vi "atm-machine.vi"() -> ()   [LabVIEW 2017]
panel:
  in  "LOGIN":bool
  out "act 6":string
  out "act 5":string
  out "act 4":string
  out "act 3":string
  out "act 1":string
  out "act 2":string
  in  "but6":bool
  in  "but5":bool
  in  "but4":bool
  in  "but3":bool
  in  "but2":bool
  in  "but1":bool
  in  "Enter PIN":string="0000"
  out "ATM Screen":string
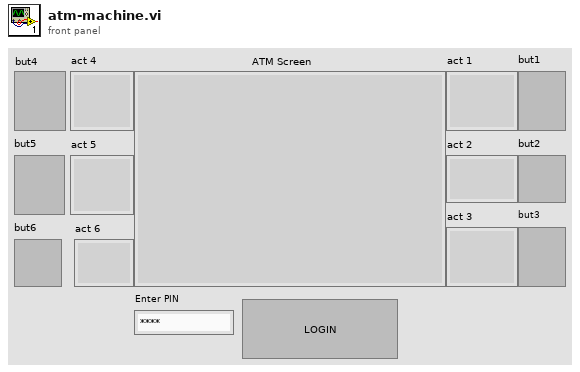
[diagram p1: front panel]
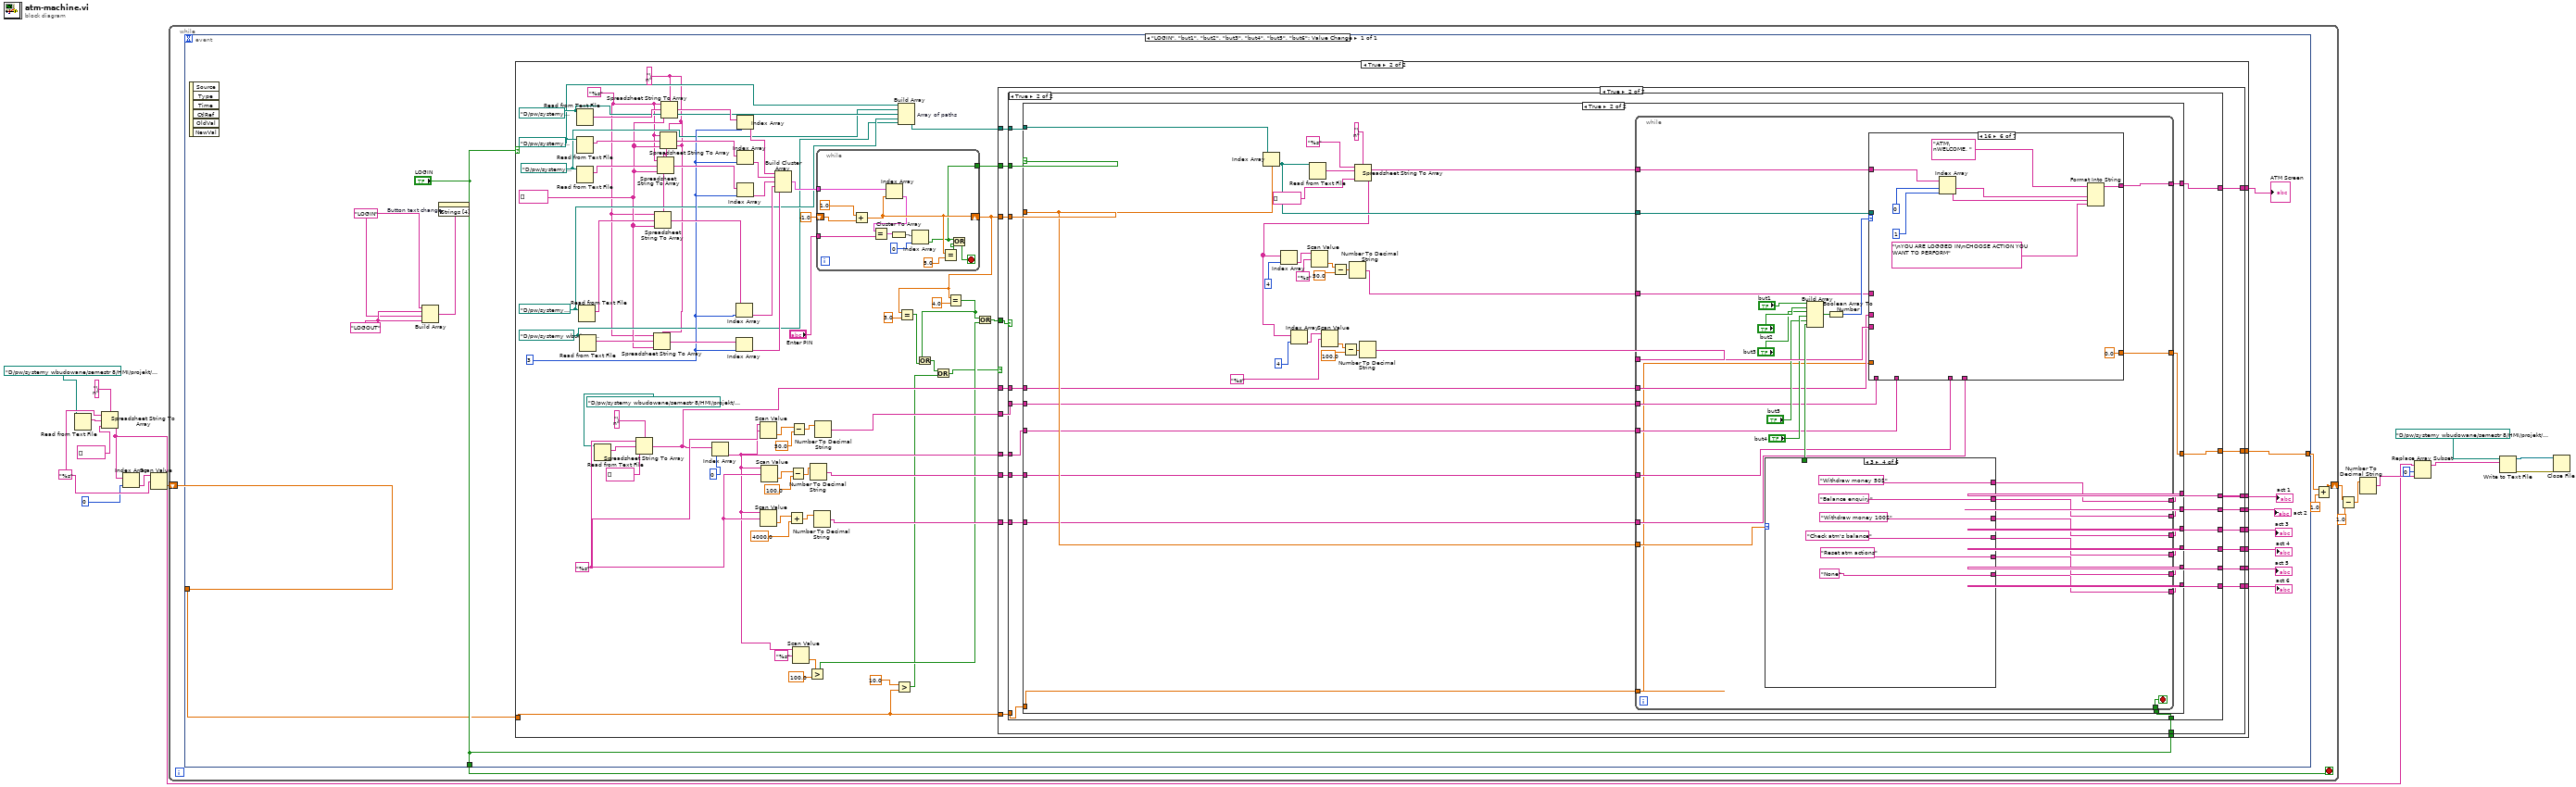
[diagram p0: block diagram]
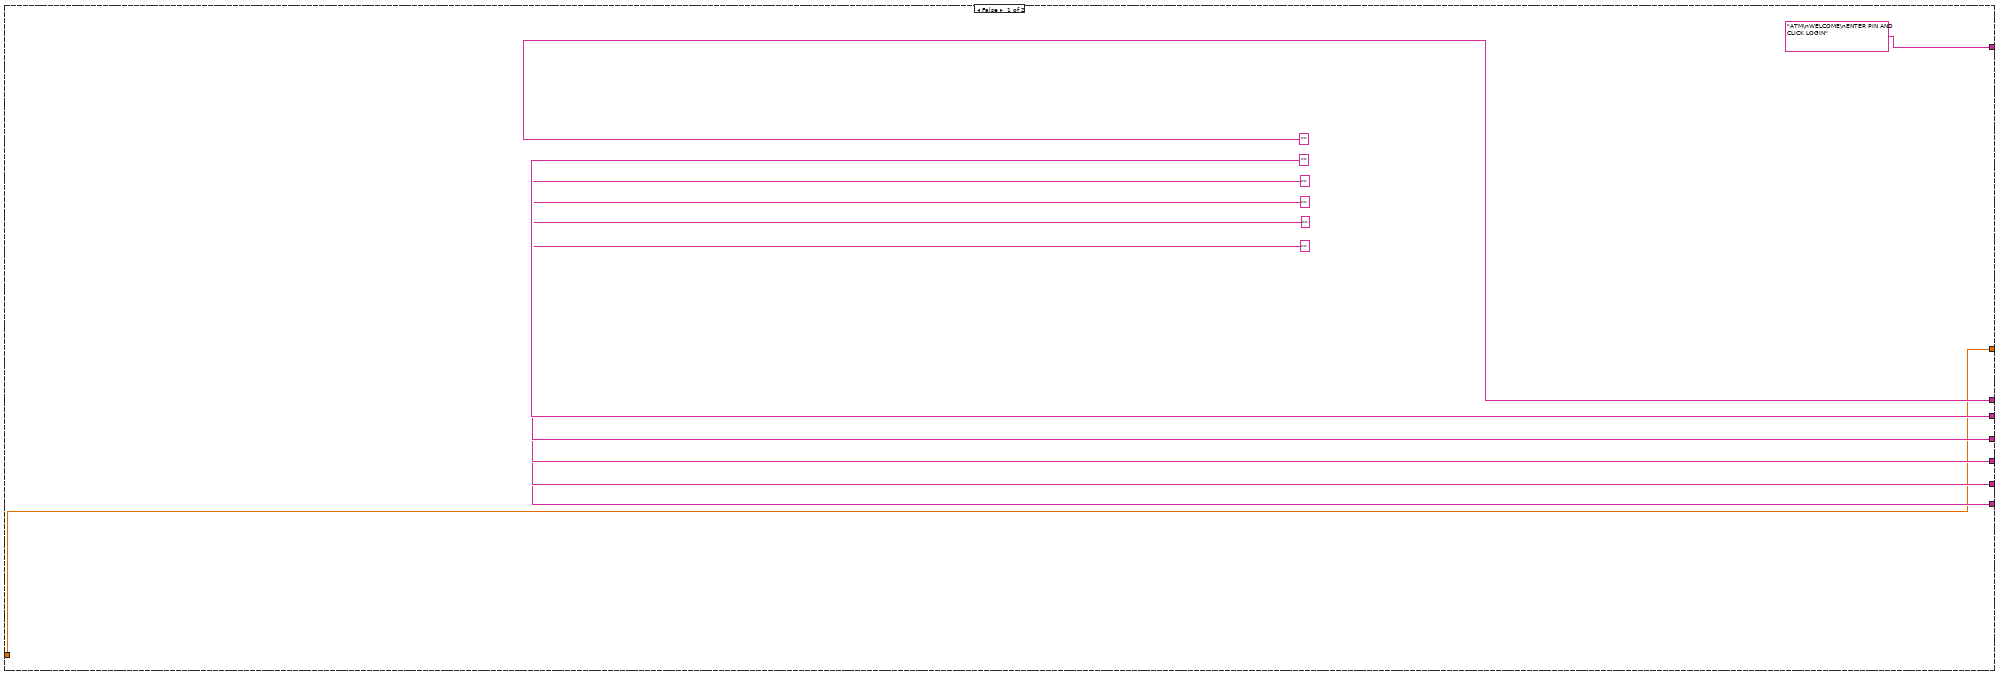
[diagram p2: hidden frame]
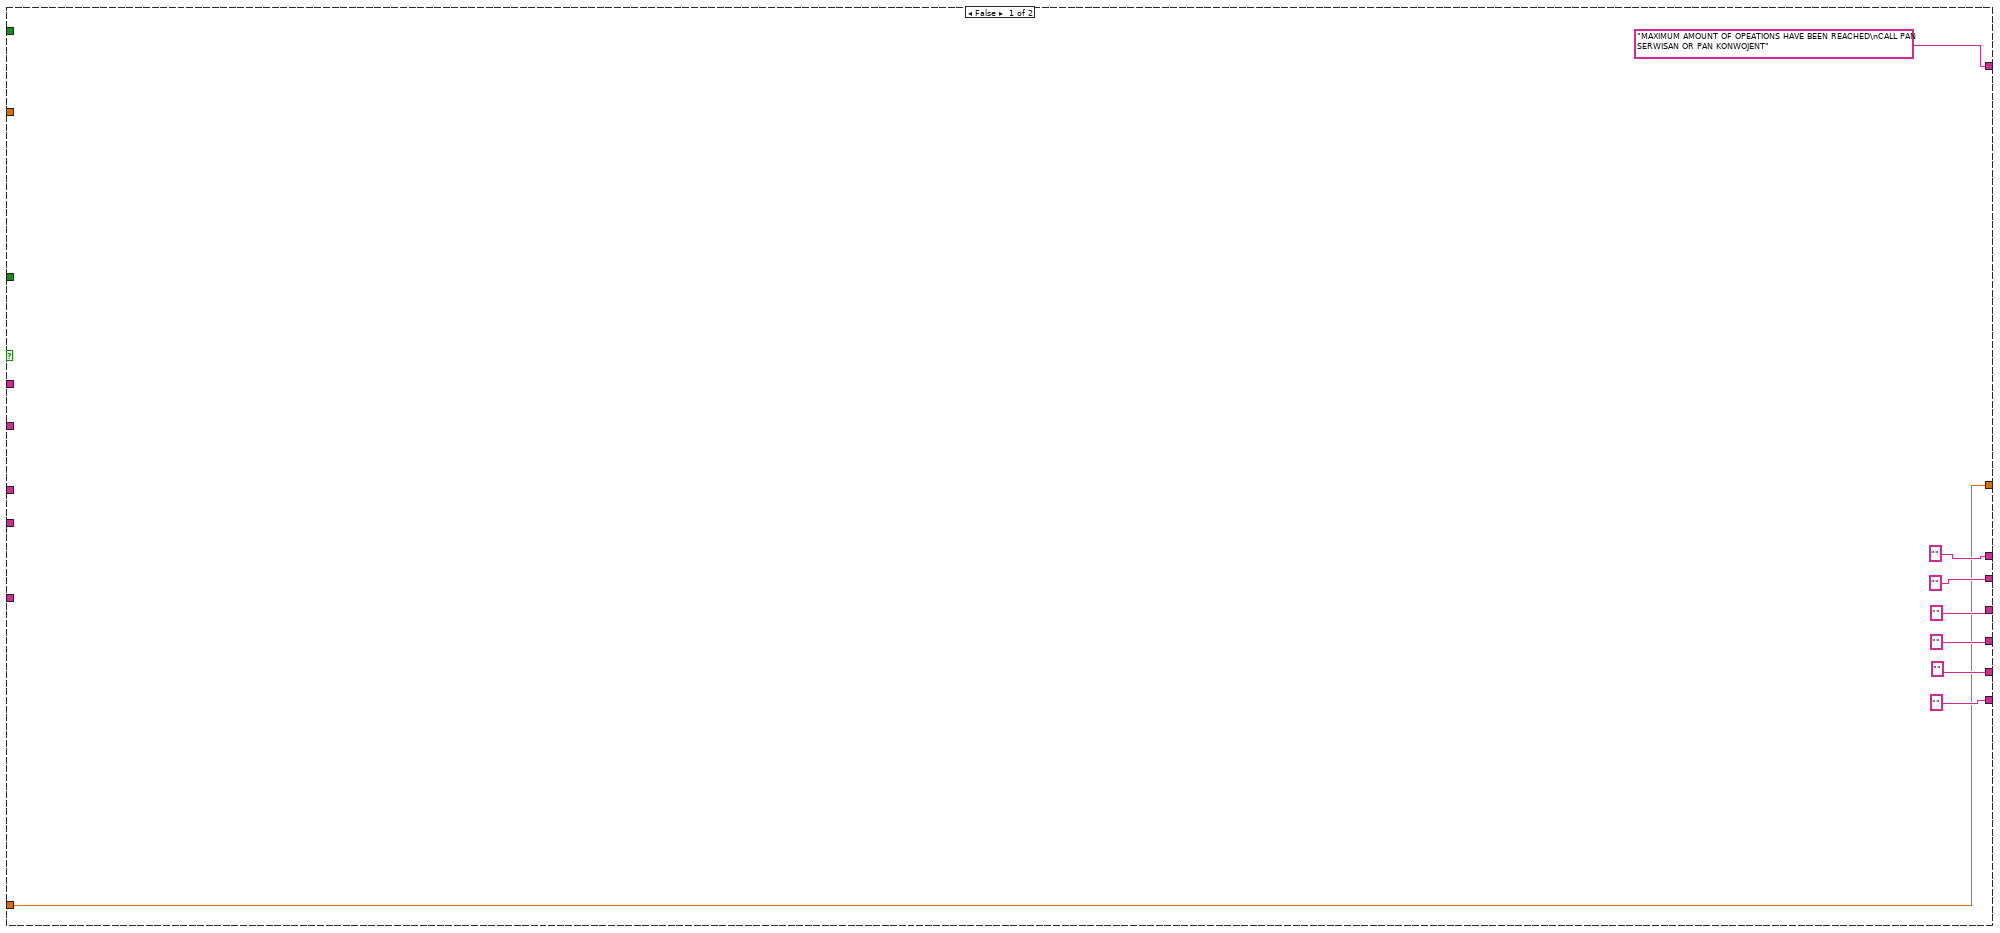
[diagram p3: hidden frame]
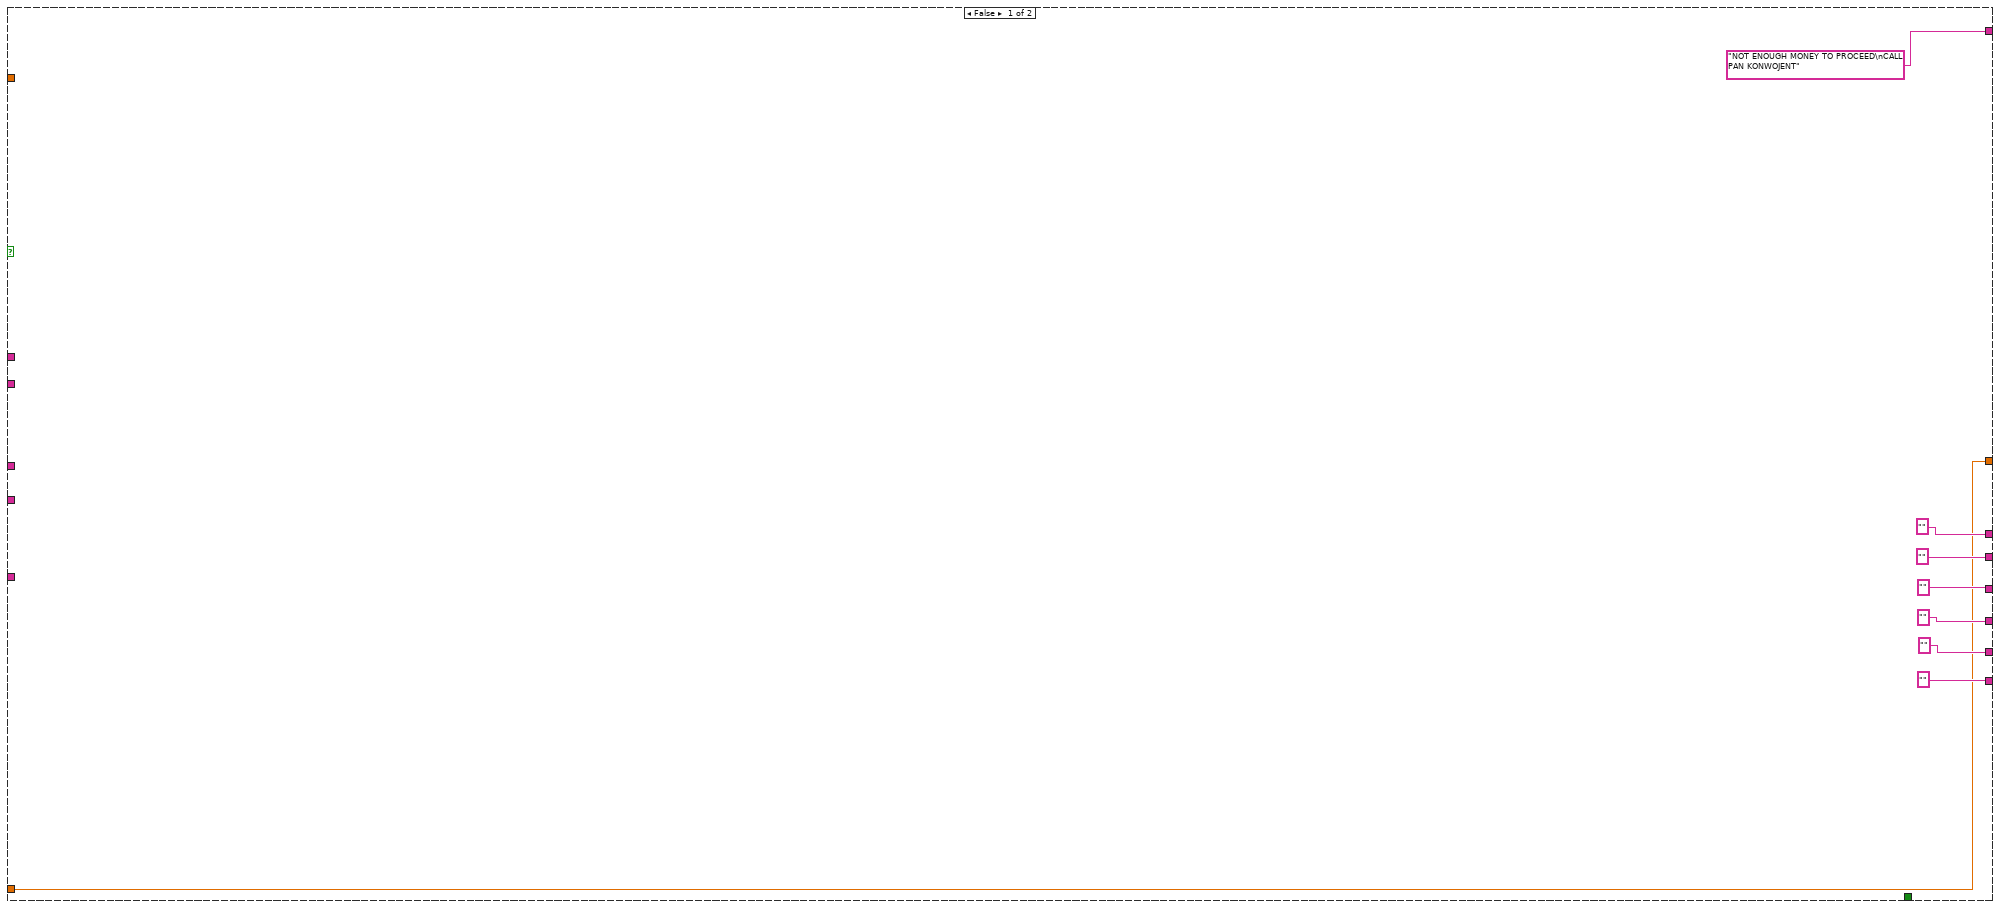
[diagram p4: hidden frame]
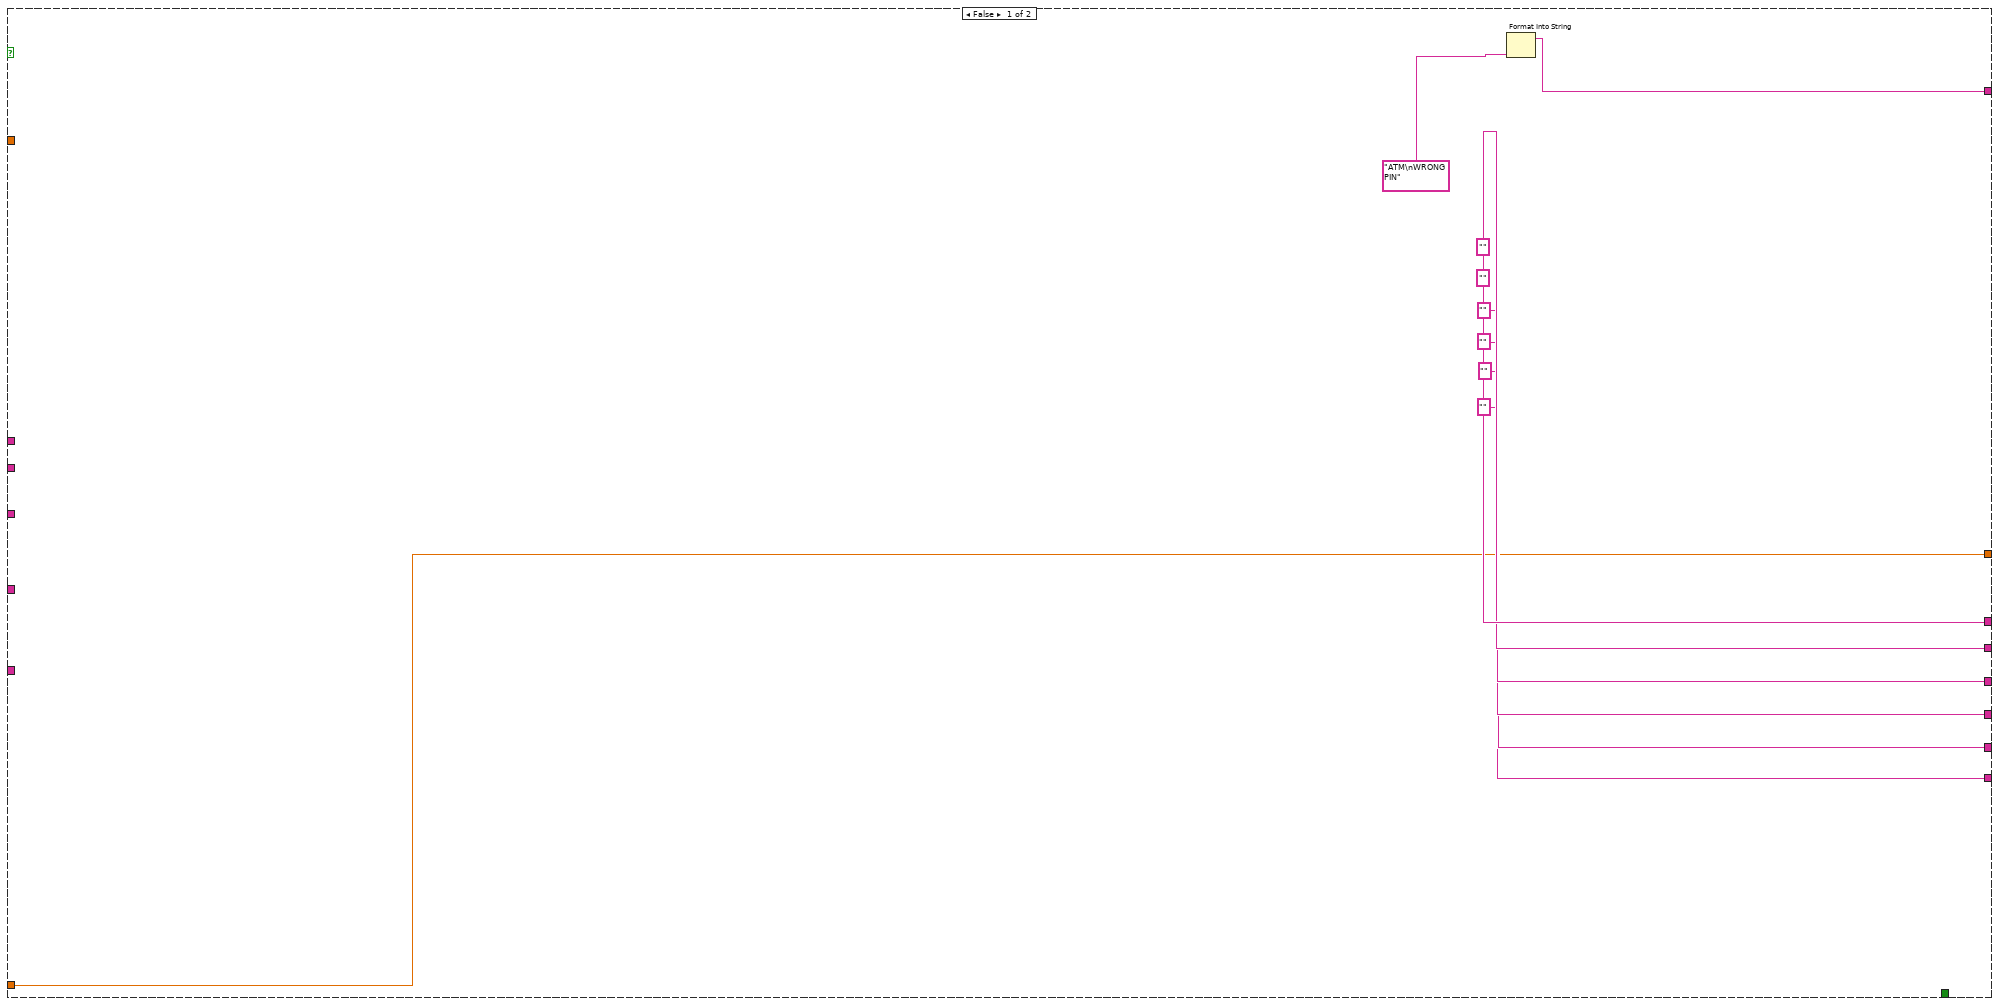
[diagram p5: hidden frame]
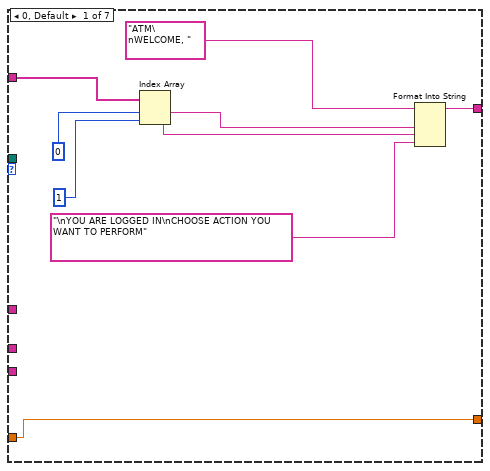
[diagram p6: hidden frame]
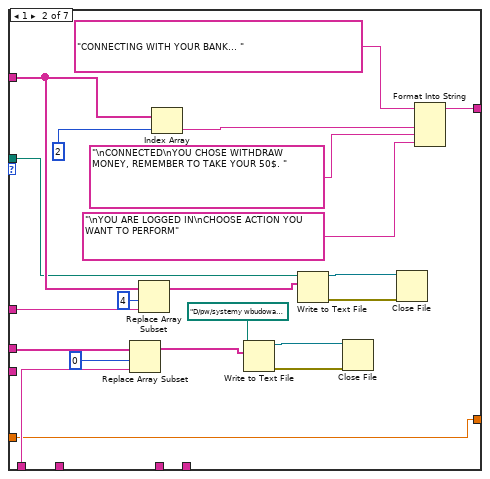
[diagram p7: hidden frame]
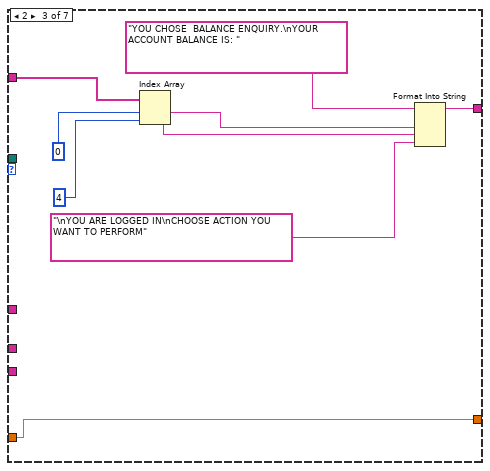
[diagram p8: hidden frame]
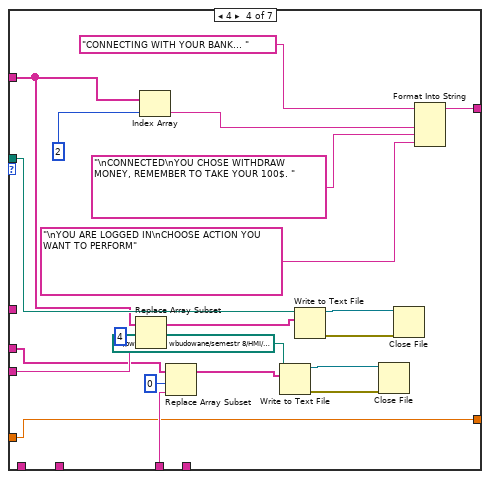
[diagram p9: hidden frame]
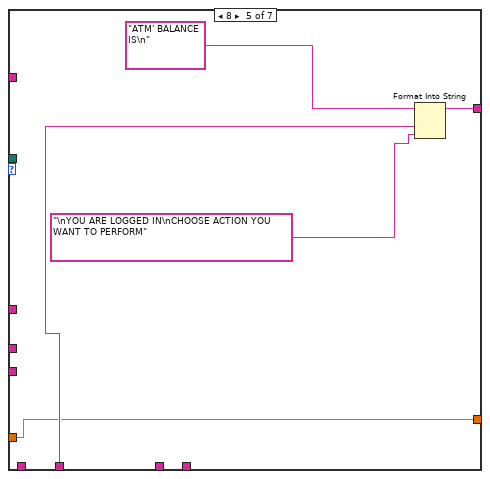
[diagram p10: hidden frame]
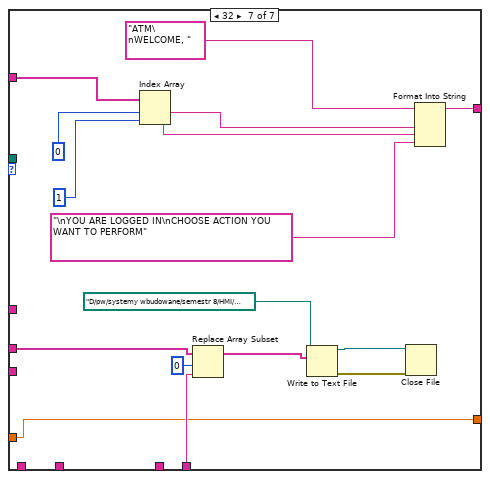
[diagram p11: hidden frame]
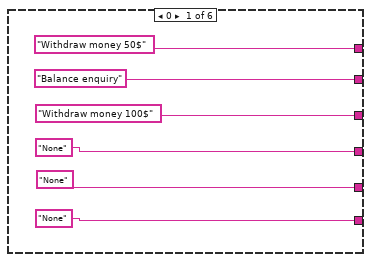
[diagram p12: hidden frame]
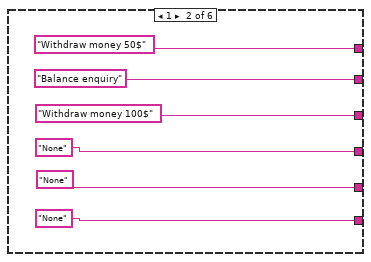
[diagram p13: hidden frame]
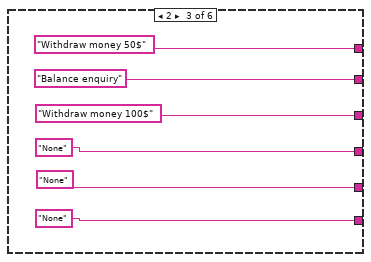
[diagram p14: hidden frame]
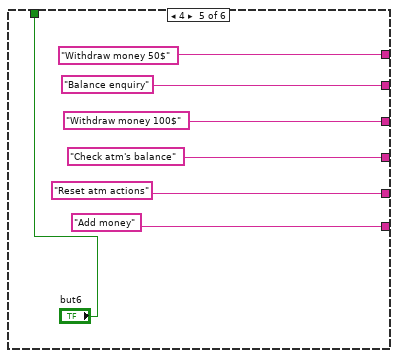
[diagram p15: hidden frame]
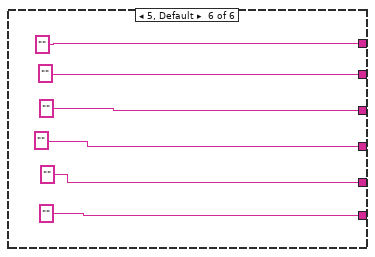
[diagram p16: hidden frame]
diagram:
  w16 = "%s" ("format string")
  n1 = Read from Text File(file (use dialog)=path "D:/pw/systemy wbudowane/semestr 8/HMI/projekt/bankomat-iteracje.txt") -> (text=w17:string)  [unwired: 3 in, 3 out]
  n2 = Spreadsheet String To Array(delimiter (Tab)="\n", format string=w16, spreadsheet string=w17, array type (2D Dbl)=string[] [] ("Array")) -> (array=w6:string[])
  n3 = Index Array "Index Array"(array=w6, index=0) -> (element=w18:string)
  n4 = Scan Value(string=w18, format string=w16) -> (value=w11:dbl)  [unwired: 1 in, 1 out]
  n5 = while {
    shift-right: [w20] -> w3
    shift-left: w11 -> [w22]
    stop <- w23 stop-if-true
    n6 = event shown="[0] \"LOGIN\", \"but1\", \"but2\", \"but3\", \"but4\", \"but5\", \"but6\": Value Change" {
      selector: _ -> [_]
      dyn-events: _ -> [_]
      timeout: _ -> [_]
      tunnel: ["LOGIN"] -> w23
      tunnel: [w25] -> w19
      tunnel: w22 -> [w24]
      event "LOGIN", "but1", "but2", "but3", "but4", "but5", "but6": Value Change {
        w29 = "LOGOUT" ("new ON text")
        w28 = "LOGIN" ("new OFF text")
        n7 = event-data() -> ()  [unwired: 1 in, 6 out]
        n8 = Build Array(w28, w29, w28, w29) -> (w30:string[])
        n9 = property on="Button text change" class="Bool (strict)"("Strings [4]"=w30) -> ()  [unwired: 2 in, 2 out]
        n10 = case shown="True" "LOGIN" {
          tunnel: ["" w93] -> w36
          tunnel: ["" w94] -> w35
          tunnel: ["" w95] -> w34
          tunnel: ["" w96] -> w33
          tunnel: ["" w98] -> w32
          tunnel: ["" w97] -> w31
          tunnel: "LOGIN" -> [_ w85]
          tunnel: ["ATM\nWELCOME\nENTER PIN AND CLICK LOGIN" w84] -> w26
          tunnel: [w37 w80] -> w25
          tunnel: w24 -> [w37 w51]
          frame False {
          }
          frame True {
            w67 = "%s" ("format string")
            w81 = "\n" ("delimiter (Tab)")
            w82 = "%s" ("format string")
            w106 = 3 ("index (row)")
            w83 = string[] [] ("Array")
            w87 = path "D:/pw/systemy wbudowane/semestr 8/HMI/projekt/konwojent.txt" ("file (use dialog)")
            w88 = path "D:/pw/systemy wbudowane/semestr 8/HMI/projekt/serwisant.txt" ("file (use dialog)")
            w89 = path "D:/pw/systemy wbudowane/semestr 8/HMI/projekt/klient-3.txt" ("file (use dialog)")
            w90 = path "D:/pw/systemy wbudowane/semestr 8/HMI/projekt/klient-2.txt" ("file (use dialog)")
            w91 = path "D:/pw/systemy wbudowane/semestr 8/HMI/projekt/klient-1.txt" ("file (use dialog)")
            n11 = Read from Text File(file (use dialog)=w90) -> (text=w114:string)  [unwired: 3 in, 3 out]
            n12 = Read from Text File(file (use dialog)=w89) -> (text=w113:string)  [unwired: 3 in, 3 out]
            n13 = Read from Text File(file (use dialog)=w91) -> (text=w117:string)  [unwired: 3 in, 3 out]
            n14 = Read from Text File(file (use dialog)=w88) -> (text=w112:string)  [unwired: 3 in, 3 out]
            n15 = Read from Text File(file (use dialog)=w87) -> (text=w111:string)  [unwired: 3 in, 3 out]
            n16 = Read from Text File(file (use dialog)=path "D:/pw/systemy wbudowane/semestr 8/HMI/projekt/bankomat-stan-konta.txt") -> (text=w78:string)  [unwired: 3 in, 3 out]
            n17 = Spreadsheet String To Array(delimiter (Tab)="\n", format string=w67, spreadsheet string=w78, array type (2D Dbl)=string[] [] ("Array")) -> (array=w61:string[])
            n18 = Spreadsheet String To Array(delimiter (Tab)=w81, format string=w82, spreadsheet string=w111, array type (2D Dbl)=w83) -> (array=w107:string[])
            n19 = Spreadsheet String To Array(delimiter (Tab)=w81, format string=w82, spreadsheet string=w112, array type (2D Dbl)=w83) -> (array=w108:string[])
            n20 = Spreadsheet String To Array(delimiter (Tab)=w81, format string=w82, spreadsheet string=w113, array type (2D Dbl)=w83) -> (array=w109:string[])
            n21 = Spreadsheet String To Array(delimiter (Tab)=w81, format string=w82, spreadsheet string=w114, array type (2D Dbl)=w83) -> (array=w110:string[])
            n22 = Spreadsheet String To Array(delimiter (Tab)=w81, format string=w82, spreadsheet string=w117, array type (2D Dbl)=w83) -> (array=w116:string[])
            n23 = Index Array "Index Array"(array=w61, index=0) -> (element=w60:string)
            n24 = Index Array "Index Array"(array=w108, index=w106) -> (element=w103:string)
            n25 = Index Array "Index Array"(array=w107, index=w106) -> (element=w102:string)
            n26 = Index Array "Index Array"(array=w109, index=w106) -> (element=w104:string)
            n27 = Index Array "Index Array"(array=w116, index=w106) -> (element=w115:string)
            n28 = Index Array "Index Array"(array=w110, index=w106) -> (element=w105:string)
            n29 = Scan Value(string=w60, format string=w67) -> (value=w74:dbl)  [unwired: 1 in, 1 out]
            n30 = Scan Value(string=w60, format string=w67) -> (value=w72:dbl)  [unwired: 1 in, 1 out]
            n31 = Scan Value(string=w60, format string=w67) -> (value=w73:dbl)  [unwired: 1 in, 1 out]
            n32 = Build Cluster Array "Build Cluster Array"(w115, w105, w104, w103, w102) -> (w101:cluster{"String":string}[])
            n33 = Add(x=w74, y=4000.0) -> (x+y=w77:dbl)
            n34 = Subtract(x=w73, y=100.0) -> (x-y=w76:dbl)
            n35 = Subtract(x=w72, y=50.0) -> (x-y=w75:dbl)
            n36 = Scan Value(string=w60, format string="%s") -> (value=w79:dbl)  [unwired: 1 in, 1 out]
            n37 = Greater?(x=w79, y=100.0) -> (0:w56:bool)
            n38 = Number To Decimal String(number=w76) -> (decimal integer string=w58:string)  [unwired: 1 in]
            n39 = Number To Decimal String(number=w77) -> (decimal integer string=w59:string)  [unwired: 1 in]
            n40 = Number To Decimal String(number=w75) -> (decimal integer string=w57:string)  [unwired: 1 in]
            n41 = while {
              tunnel: w101 -> [w384]
              shift-right: [w380] -> w53
              shift-left: -1.0 -> [w382]
              tunnel: "Enter PIN" -> [w379]
              tunnel: [w372] -> w92
              stop <- w373 stop-if-true
              n42 = Add(x=1.0 ("y"), y=w382) -> (x+y=w380:dbl)
              n43 = Index Array "Index Array"(array=w384, index=w380) -> (element=w378:cluster{"String":string})
              n44 = Equal?(x=w378, y=w379) -> (x = y?=w377:cluster{"String":bool})
              n45 = Cluster To Array(cluster=w377) -> (array=w376:bool[])
              n46 = Index Array "Index Array"(array=w376, index=0) -> (element=w372:bool)
              n47 = Equal?(x=w380, y=5.0 ("x")) -> (x = y?=w374:bool)
              n48 = Or(x=w372, y=w374) -> (x .or. y?=w373:bool)
            }
            n49 = Greater?(x=10.0, y=w51) -> (0:w49:bool)
            n50 = Build Array "Array of paths"(w91, w90, w89, w88, w87) -> (w86:path[])
            n51 = Equal?(x=w53, y=3.0) -> (x = y?=w46:bool)
            n52 = Equal?(x=w53, y=4.0) -> (x = y?=w45:bool)
            n53 = Or(x=w45, y=w46) -> (x .or. y?=w47:bool)
            n54 = Or(x=w47, y=w49) -> (x .or. y?=w48:bool)
            n55 = Or(x=w45, y=w56) -> (x .or. y?=w55:bool)
            n56 = case shown="True" w48 {
              tunnel: ["" w144] -> w98
              tunnel: ["" w143] -> w97
              tunnel: ["" w142] -> w96
              tunnel: ["" w141] -> w95
              tunnel: ["" w140] -> w94
              tunnel: ["" w139] -> w93
              tunnel: w92 -> [_ w138]
              tunnel: w86 -> [_ w137]
              tunnel: w85 -> [_ w136]
              tunnel: ["MAXIMUM AMOUNT OF OPEATIONS HAVE BEEN REACHED\nCALL PAN SERWISAN OR PAN KONWOJENT" w135] -> w84
              tunnel: [w118 w134] -> w80
              tunnel: w61 -> [_ w133]
              tunnel: w60 -> [_ w132]
              tunnel: w59 -> [_ w131]
              tunnel: w58 -> [_ w130]
              tunnel: w57 -> [_ w129]
              tunnel: w55 -> [_ w128]
              tunnel: w53 -> [_ w127]
              tunnel: w51 -> [w118 w126]
              frame False {
              }
              frame True {
                n57 = case shown="True" w128 {
                  tunnel: ["" w170] -> w144
                  tunnel: ["" w169] -> w143
                  tunnel: ["" w168] -> w142
                  tunnel: ["" w167] -> w141
                  tunnel: ["" w166] -> w140
                  tunnel: ["" w165] -> w139
                  tunnel: w138 -> [_ w164]
                  tunnel: w127 -> [_ w163]
                  tunnel: w137 -> [_ w162]
                  tunnel: w136 -> [_ w161]
                  tunnel: ["NOT ENOUGH MONEY TO PROCEED\nCALL PAN KONWOJENT" w160] -> w135
                  tunnel: [w145 w159] -> w134
                  tunnel: w126 -> [w145 w158]
                  tunnel: w133 -> [_ w157]
                  tunnel: w132 -> [_ w156]
                  tunnel: w131 -> [_ w155]
                  tunnel: w130 -> [_ w154]
                  tunnel: w129 -> [_ w153]
                  frame False {
                  }
                  frame True {
                    n58 = case shown="True" w164 {
                      tunnel: ["" w216] -> w170
                      tunnel: ["" w214] -> w169
                      tunnel: ["" w215] -> w168
                      tunnel: ["" w213] -> w167
                      tunnel: ["" w212] -> w166
                      tunnel: ["" w211] -> w165
                      tunnel: w163 -> [_ w210]
                      tunnel: w162 -> [_ w196]
                      tunnel: [w172 w209] -> w160
                      tunnel: w161 -> [_ w208]
                      tunnel: [w171 w180] -> w159
                      tunnel: w158 -> [w171 w187]
                      tunnel: w157 -> [_ w185]
                      tunnel: w156 -> [_ w184]
                      tunnel: w155 -> [_ w183]
                      tunnel: w154 -> [_ w182]
                      tunnel: w153 -> [_ w181]
                      frame False {
                        n59 = Format Into String("ATM\nWRONG PIN") -> (resulting string=w172:string)  [unwired: 3 in, 1 out]
                      }
                      frame True {
                        n60 = Index Array "Index Array"(array=w196, index=w210) -> (element=w195:path)
                        n61 = Read from Text File(file (use dialog)=w195) -> (text=w207:string)  [unwired: 3 in, 3 out]
                        n62 = Spreadsheet String To Array(delimiter (Tab)="\n", format string="%s", spreadsheet string=w207, array type (2D Dbl)=string[] [] ("Array")) -> (array=w190:string[])
                        n63 = Index Array "Index Array"(array=w190, index=4 ("disabled index (col)")) -> (element=w204:string)
                        n64 = Index Array "Index Array"(array=w190, index=4 ("disabled index (col)")) -> (element=w194:string)
                        n65 = Scan Value(string=w204, format string="%s") -> (value=w203:dbl)  [unwired: 1 in, 1 out]
                        n66 = Scan Value(string=w194, format string="%s") -> (value=w193:dbl)  [unwired: 1 in, 1 out]
                        n67 = Subtract(x=w203, y=50.0) -> (x-y=w201:dbl)
                        n68 = Subtract(x=w193, y=100.0) -> (x-y=w191:dbl)
                        n69 = Number To Decimal String(number=w201) -> (decimal integer string=w198:string)  [unwired: 1 in]
                        n70 = Number To Decimal String(number=w191) -> (decimal integer string=w188:string)  [unwired: 1 in]
                        n71 = while {
                          tunnel: [w244] -> w216
                          tunnel: [w243] -> w215
                          tunnel: [w242] -> w214
                          tunnel: [w241] -> w213
                          tunnel: [w240] -> w212
                          tunnel: [w239] -> w211
                          tunnel: w210 -> [w238]
                          tunnel: [w237] -> w209
                          tunnel: w208 -> [w230]
                          tunnel: w190 -> [w229]
                          tunnel: w198 -> [w228]
                          tunnel: w195 -> [w227]
                          tunnel: w188 -> [w226]
                          tunnel: w187 -> [w218]
                          tunnel: w185 -> [w223]
                          tunnel: w184 -> [w222]
                          tunnel: w183 -> [w221]
                          tunnel: w182 -> [w220]
                          tunnel: w181 -> [w219]
                          tunnel: [w217] -> w180
                          stop <- w230 stop-if-true
                          n72 = case shown="3" w238 {
                            tunnel: ["Withdraw money 50$" "Withdraw money 50$" "Withdraw money 50$" "Withdraw money 50$" "Withdraw money 50$" ""] -> w244
                            tunnel: ["Withdraw money 100$" "Withdraw money 100$" "Withdraw money 100$" "Withdraw money 100$" "Withdraw money 100$" ""] -> w243
                            tunnel: ["Balance enquiry" "Balance enquiry" "Balance enquiry" "Balance enquiry" "Balance enquiry" ""] -> w242
                            tunnel: ["None" "None" "None" "Check atm's balance" "Check atm's balance" ""] -> w241
                            tunnel: ["None" "None" "None" "Reset atm actions" "Reset atm actions" ""] -> w240
                            tunnel: ["None" "None" "None" "None" "Add money" ""] -> w239
                            tunnel: [_ _ _ _ "but6" _] -> w232
                            frame 0 {
                            }
                            frame 1 {
                            }
                            frame 2 {
                            }
                            frame 3 {
                            }
                            frame 4 {
                            }
                            frame 5, Default {
                            }
                          }
                          n73 = Build Array("but1", "but2", "but3", "but4", "but5", w232) -> (w233:bool[])
                          n74 = Boolean Array To Number(Boolean array=w233) -> (number=w231:u32)
                          n75 = case shown="16" w231 {
                            tunnel: [w253 w274 w283 w304 w309 w318 w334] -> w237
                            tunnel: w229 -> [w252 w269 w282 w295 _ w317 w333]
                            tunnel: w228 -> [_ w268 _ _ _ _ _]
                            tunnel: w227 -> [_ w266 _ w296 _ _ _]
                            tunnel: w226 -> [_ _ _ w294 _ _ _]
                            tunnel: w222 -> [_ _ _ _ w306 _ _]
                            tunnel: w219 -> [_ w261 _ _ _ _ _]
                            tunnel: w223 -> [_ w260 _ w286 _ _ w321]
                            tunnel: w220 -> [_ _ _ w285 _ _ _]
                            tunnel: w221 -> [_ _ _ _ _ _ w320]
                            tunnel: w218 -> [w245 w254 w275 w284 w305 _ w319]
                            tunnel: [w245 w254 w275 w284 w305 0.0 w319] -> w217
                            frame 0, Default {
                              n76 = Index Array "Index Array"(array=w252, index #1=0 ("index (row)"), index #2=1 ("disabled index (row)")) -> (element #1=w248:string, element #2=w247:string)
                              n77 = Format Into String(initial string="ATM\nWELCOME, ", w248, w247, "\nYOU ARE LOGGED IN\nCHOOSE ACTION YOU WANT TO PERFORM") -> (resulting string=w253:string)  [unwired: 2 in, 1 out]
                            }
                            frame 1 {
                              n78 = Replace Array Subset "Replace Array Subset"(array=w260, new element=w261, index=0) -> (w256:string[])
                              n79 = Replace Array Subset "Replace Array Subset"(array=w269, new element=w268, index=4) -> (w265:string[])
                              n80 = Index Array "Index Array"(array=w269, index=2 ("index (row)")) -> (element=w271:string)
                              n81 = Write to Text File(file (use dialog)=path "D:/pw/systemy wbudowane/semestr 8/HMI/projekt/bankomat-stan-konta.txt", text=w256) -> (refnum out=w258:refnum<file>, error out=w257:errorcluster)  [unwired: 2 in, 1 out]
                              n82 = Write to Text File(file (use dialog)=w266, text=w265) -> (refnum out=w264:refnum<file>, error out=w263:errorcluster)  [unwired: 2 in, 1 out]
                              n83 = Close File(refnum=w258, error in=w257) -> ()  [unwired: 2 out]
                              n84 = Close File(refnum=w264, error in=w263) -> ()  [unwired: 2 out]
                              n85 = Format Into String(initial string="CONNECTING WITH YOUR BANK... ", w271, "\nCONNECTED\nYOU CHOSE WITHDRAW MONEY, REMEMBER TO TAKE YOUR 50$. ", "\nYOU ARE LOGGED IN\nCHOOSE ACTION YOU WANT TO PERFORM") -> (resulting string=w274:string)  [unwired: 2 in, 1 out]
                            }
                            frame 2 {
                              n86 = Index Array "Index Array"(array=w282, index #1=0 ("index (row)"), index #2=4 ("disabled index (row)")) -> (element #1=w278:string, element #2=w277:string)
                              n87 = Format Into String(initial string="YOU CHOSE  BALANCE ENQUIRY.\nYOUR ACCOUNT BALANCE IS: ", w278, w277, "\nYOU ARE LOGGED IN\nCHOOSE ACTION YOU WANT TO PERFORM") -> (resulting string=w283:string)  [unwired: 2 in, 1 out]
                            }
                            frame 4 {
                              n88 = Replace Array Subset "Replace Array Subset"(array=w295, new element=w294, index=4) -> (w299:string[])
                              n89 = Index Array "Index Array"(array=w295, index=2 ("index (row)")) -> (element=w302:string)
                              n90 = Replace Array Subset "Replace Array Subset"(array=w286, new element=w285, index=0) -> (w288:string[])
                              n91 = Write to Text File(file (use dialog)=path "D:/pw/systemy wbudowane/semestr 8/HMI/projekt/bankomat-stan-konta.txt", text=w288) -> (refnum out=w290:refnum<file>, error out=w289:errorcluster)  [unwired: 2 in, 1 out]
                              n92 = Write to Text File(file (use dialog)=w296, text=w299) -> (refnum out=w298:refnum<file>, error out=w297:errorcluster)  [unwired: 2 in, 1 out]
                              n93 = Close File(refnum=w290, error in=w289) -> ()  [unwired: 2 out]
                              n94 = Close File(refnum=w298, error in=w297) -> ()  [unwired: 2 out]
                              n95 = Format Into String(initial string="CONNECTING WITH YOUR BANK... ", w302, "\nCONNECTED\nYOU CHOSE WITHDRAW MONEY, REMEMBER TO TAKE YOUR 100$. ", "\nYOU ARE LOGGED IN\nCHOOSE ACTION YOU WANT TO PERFORM") -> (resulting string=w304:string)  [unwired: 2 in, 1 out]
                            }
                            frame 8 {
                              n96 = Format Into String(initial string="ATM' BALANCE IS\n", w306, "\nYOU ARE LOGGED IN\nCHOOSE ACTION YOU WANT TO PERFORM") -> (resulting string=w309:string)  [unwired: 2 in, 1 out]
                            }
                            frame 16 {
                              n97 = Index Array "Index Array"(array=w317, index #1=0 ("index (row)"), index #2=1 ("disabled index (row)")) -> (element #1=w313:string, element #2=w312:string)
                              n98 = Format Into String(initial string="ATM\nWELCOME, ", w313, w312, "\nYOU ARE LOGGED IN\nCHOOSE ACTION YOU WANT TO PERFORM") -> (resulting string=w318:string)  [unwired: 2 in, 1 out]
                            }
                            frame 32 {
                              n99 = Index Array "Index Array"(array=w333, index #1=0 ("index (row)"), index #2=1 ("disabled index (row)")) -> (element #1=w329:string, element #2=w328:string)
                              n100 = Replace Array Subset "Replace Array Subset"(array=w321, new element=w320, index=0) -> (w323:string[])
                              n101 = Write to Text File(file (use dialog)=path "D:/pw/systemy wbudowane/semestr 8/HMI/projekt/bankomat-stan-konta.txt", text=w323) -> (refnum out=w325:refnum<file>, error out=w324:errorcluster)  [unwired: 2 in, 1 out]
                              n102 = Close File(refnum=w325, error in=w324) -> ()  [unwired: 2 out]
                              n103 = Format Into String(initial string="ATM\nWELCOME, ", w329, w328, "\nYOU ARE LOGGED IN\nCHOOSE ACTION YOU WANT TO PERFORM") -> (resulting string=w334:string)  [unwired: 2 in, 1 out]
                            }
                          }
                        }
                      }
                    }
                  }
                }
              }
            }
          }
        }
        "act 2" <- w31
        "act 1" <- w32
        "act 3" <- w33
        "act 4" <- w34
        "act 5" <- w35
        "act 6" <- w36
        "ATM Screen" <- w26
      }
    }
    n104 = Add(x=w19, y=1.0) -> (x+y=w20:dbl)
  }
  n105 = Subtract(x=w3, y=1.0) -> (x-y=w2:dbl)
  n106 = Number To Decimal String(number=w2) -> (decimal integer string=w8:string)  [unwired: 1 in]
  n107 = Replace Array Subset "Replace Array Subset"(array=w6, new element=w8, index=0) -> (w5:string[])
  n108 = Write to Text File(file (use dialog)=path "D:/pw/systemy wbudowane/semestr 8/HMI/projekt/bankomat-iteracje.txt", text=w5) -> (refnum out=w10:refnum<file>, error out=w9:errorcluster)  [unwired: 2 in, 1 out]
  n109 = Close File(refnum=w10, error in=w9) -> ()  [unwired: 2 out]
